vi "Interpolate from 2 arrays.vi"(9 "Target X":dbl, 10 "Y Array":dbl[](array[numeric]), 11 "X Array":dbl[](array[numeric])) -> (3 "Interpolated Y":dbl)   [LabVIEW 2009]
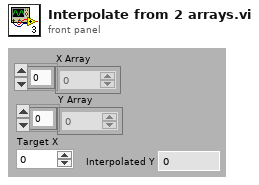
[diagram p1: front panel]
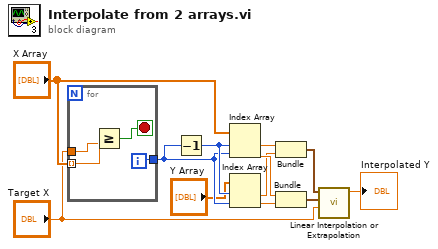
[diagram p0: block diagram]
diagram:
  n1 = for {
    tunnel: "X Array" -> [w16] mode=indexing
    tunnel: "Target X" -> [w15]
    tunnel: [w13] -> w5
    i -> [w13]
    stop <- w14 stop-if-true
    n2 = Greater Or Equal?(x=w16, y=w15) -> (x >= y?=w14:bool)
  }
  n3 = Decrement(x=w5) -> (x-1=w7:i32)
  n4 = Index Array(array="X Array", index #1=w7, index #2=w5) -> (element #1=w8:dbl, element #2=w10:dbl)
  n5 = Index Array(array="Y Array", index #1=w7, index #2=w5) -> (element #1=w9:dbl, element #2=w11:dbl)
  n6 = Bundle(w8, w9) -> (w6:cluster{dbl, dbl})  [unwired: 1 in]
  n7 = Bundle(w10, w11) -> (w12:cluster{dbl, dbl})  [unwired: 1 in]
  n8 = call "Linear Interpolation or Extrapolation.vi"("X"="Target X", "Point 2"=w12, "Point 1"=w6) -> ("Y"=→"Interpolated Y":dbl)  [unwired: 8 in]
